vi "SMAC.vi"() -> ()   [LabVIEW 2023]
uses:
  <vilib>/Instr/_visa.llb/VISA Configure Serial Port (Instr).vi
panel:
  out "read buffer":string
  out "return count":u32
  out "error out":errorcluster
  in  "write buffer":string
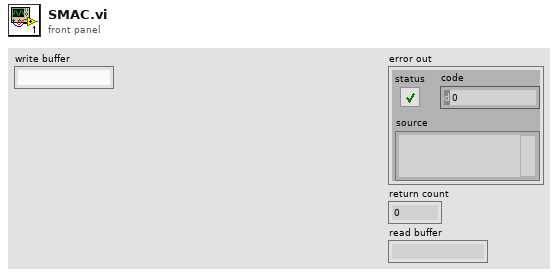
[diagram p1: front panel]
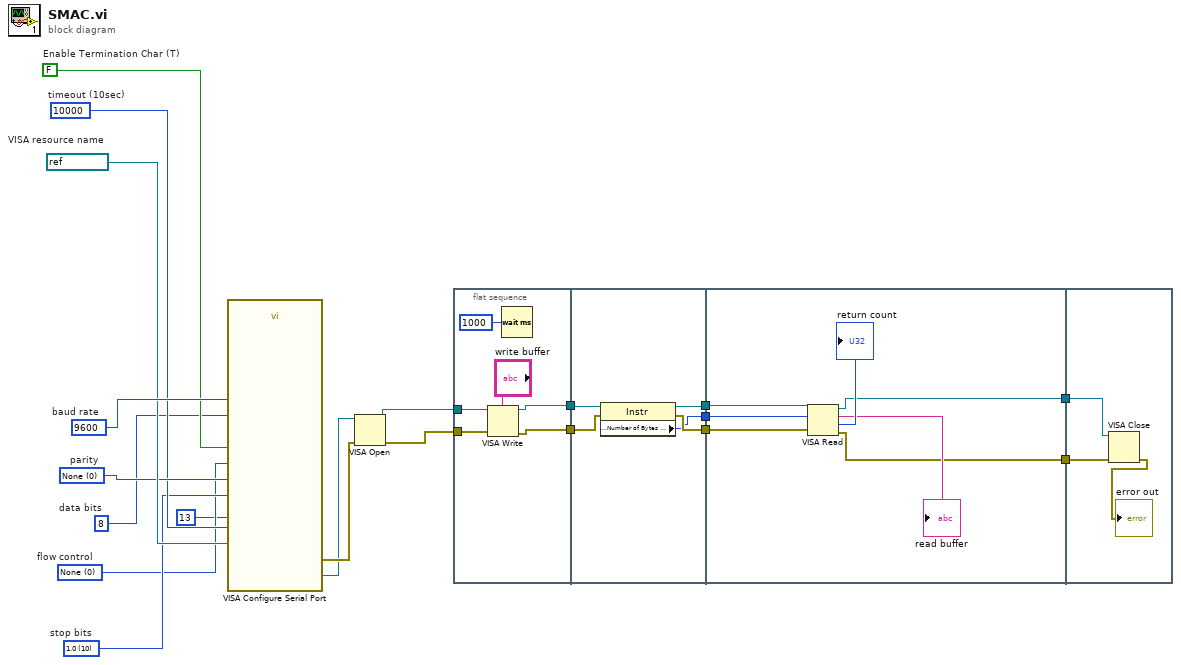
[diagram p0: block diagram]
diagram:
  w19 = refnum<visa-resource-name> "COM4"  # VISA resource name
  w20 = u32 9600  # baud rate
  w14 = u16 0 items=["None"=0, "XON/XOFF"=1, "RTS/CTS"=2, "DTR/DSR"=4]  # flow control
  w15 = u16 10 items=["1.0"=10, "1.5"=15, "2.0"=20]  # stop bits
  w18 = u16 0 items=["None", "Odd", "Even", "Mark", "Space"]  # parity
  w13 = u16 8  # data bits
  w16 = FALSE  # Enable Termination Char (T)
  w17 = u32 10000  # timeout (10sec)
  n1 = call-poly "VISA Configure Serial Port"("VISA resource name"=w19, "timeout (10sec)"=w17, "termination char\n(0xA = '\\n' = LF)"=u8 13 ("termination char\n(0xA = '\\n' = LF)"), "Enable Termination\nChar (T)"=w16, "baud rate (9600)"=w20, "data bits (8)"=w13, "parity (0:none)"=w18, "stop bits (10: 1 bit)"=w15, "flow control (0:none)"=w14) -> ("VISA resource name out"=w10:refnum<visa-resource-name>, "error out"=w11:errorcluster)  [unwired: 5 in]
  n2 = VISA Open(error in (no error)=w11, VISA resource name=w10) -> (VISA resource name=w9:refnum<visa-resource-name>, error out=w8:errorcluster)  [unwired: 3 in]
  n3 = flat-sequence {
    tunnel: w9 -> [w25]
    tunnel: w8 -> [w24]
    tunnel: [w22] -> w7
    tunnel: [w21] -> w6
    tunnel: w7 -> [w30]
    tunnel: w6 -> [w31]
    tunnel: [w28] -> w5
    tunnel: [w29] -> w4
    tunnel: [w27] -> w3
    tunnel: w5 -> [w38]
    tunnel: w4 -> [w37]
    tunnel: w3 -> [w34]
    tunnel: [w33] -> w2
    tunnel: [w32] -> w1
    tunnel: w2 -> [w40]
    tunnel: w1 -> [w39]
    frame #0 {
      n4 = VISA Write(VISA resource name=w25, write buffer="write buffer", error in (no error)=w24) -> (VISA resource name out=w21:refnum<visa-resource-name>, error out=w22:errorcluster)  [unwired: 1 out]
      n5 = Wait (ms)(milliseconds to wait=u32 1000) -> ()  [unwired: 1 out]
    }
    frame #1 {
      n6 = property class="Instr"(reference=w31, error in=w30) -> (reference out=w29:refnum<visa-resource-name>, error out=w28:errorcluster, "Serial Settings:Number of Bytes at Serial Port"=w27:u32)
    }
    frame #2 {
      n7 = VISA Read(VISA resource name=w37, byte count=w34, error in (no error)=w38) -> (VISA resource name out=w33:refnum<visa-resource-name>, read buffer=→"read buffer":string, return count=→"return count":u32, error out=w32:errorcluster)
    }
    frame #3 {
      n8 = VISA Close(VISA resource name=w40, error in (no error)=w39) -> (error out=→"error out":errorcluster)
    }
  }
